vi "Collision Detection.vi"(10 "Collision Threshold":dbl=0.5) -> (3 "Colision Detected":bool)   [LabVIEW 2017]
uses:
  <vilib>/Rock Robotics/Network Tables/SD Write Boolean.vi
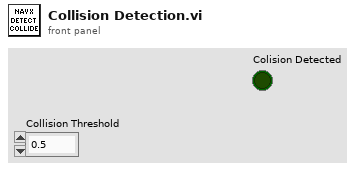
[diagram p1: front panel]
types:
  T1 = cluster{"LinearAcceleration X":dbl, "LinearAcceleration Y":dbl, "LinearAcceleration Z":dbl}
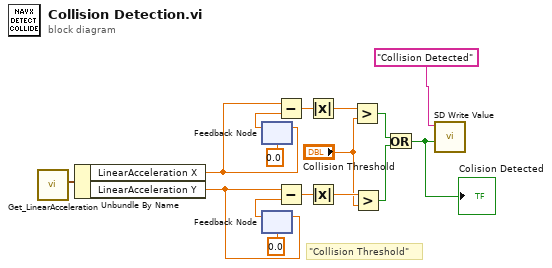
[diagram p0: block diagram]
diagram:
  # "\"Collision Threshold\""
  n1 = call <vilib>:"Get_LinearAcceleration.vi"() -> ("Linear Acceleration"=w4:T1)  [unwired: 11 in]
  n2 = Unbundle By Name(w4) -> ("LinearAcceleration X"=w12:dbl, "LinearAcceleration Y"=w5:dbl)
  n3 = feedback #1(0.0) -> (w13:dbl)
  n4 = feedback-in #1(w12) -> ()
  n5 = feedback #2(0.0) -> (w11:dbl)
  n6 = feedback-in #2(w5) -> ()
  n7 = Subtract(x=w12, y=w13) -> (x-y=w15:dbl)
  n8 = Subtract(x=w5, y=w11) -> (x-y=w9:dbl)
  n9 = Absolute Value(x=w15) -> (abs(x)=w14:dbl)
  n10 = Absolute Value(x=w9) -> (abs(x)=w10:dbl)
  n11 = Greater?(x=w14, y="Collision Threshold") -> (0:w7:bool)
  n12 = Greater?(x=w10, y="Collision Threshold") -> (0:w6:bool)
  n13 = Or(x=w7, y=w6) -> (x .or. y?=w2:bool)
  "Colision Detected" <- w2
  n14 = call-poly <vilib>:"SD Write Value.vi"("Boolean"=w2, "Name"="Collision Detected") -> ()  [unwired: 8 in, 2 out]
